vi "Priority Push.vi"(8 "error in (no error)":errorcluster, 10 "Action":T1, 11 "Subsystem in":refnum<queue>) -> (0 "error out":errorcluster, 3 "Subsystem out":refnum<queue>)   [LabVIEW 2014]
uses:
  Action/Action.ctl
  Action/Action Name.ctl
panel:
  out "Interrupted?":bool
  out "Ignored?":bool
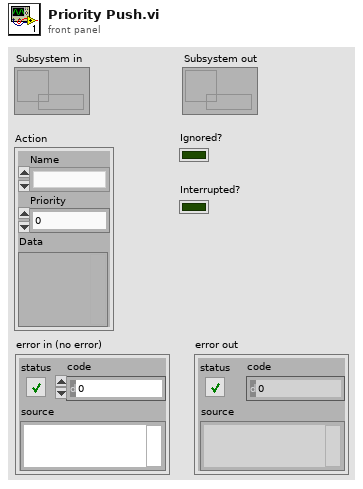
[diagram p1: front panel]
types:
  T1 = typedef "Action.ctl" = cluster{"Name":T2, "Priority":i32, "Data":variant}
  T2 = typedef "Action Name.ctl" = enum16{""}
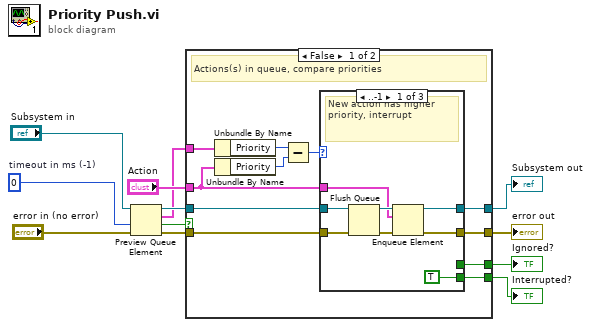
[diagram p0: block diagram]
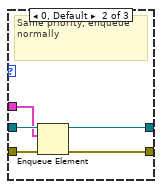
[diagram p2: hidden frame]
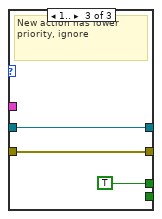
[diagram p3: hidden frame]
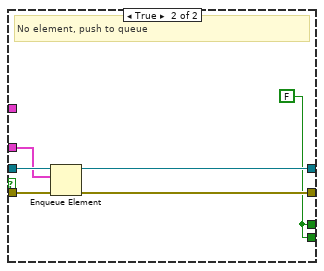
[diagram p4: hidden frame]
diagram:
  w11 = 0  # timeout in ms (-1)
  n1 = Preview Queue Element(queue="Subsystem in", timeout in ms (-1)=w11, error in (no error)="error in (no error)") -> (queue out=w9:refnum<queue>, element=w1:T1, timed out?=w10:bool, error out=w5:errorcluster)
  n2 = case shown="False" w10 {
    tunnel: w9 -> [w19 w45]
    tunnel: [w17 w44] -> w8
    tunnel: "Action" -> [w15 w43]
    tunnel: w5 -> [w18 w42]
    tunnel: [w16 w41] -> w4
    tunnel: [w14 w40] -> w3
    tunnel: [w13 w40] -> w2
    tunnel: w1 -> [w23 _]
    frame False {
      # "Actions(s) in queue, compare priorities"
      n3 = Unbundle By Name(w23) -> ("Priority"=w22:i32)
      n4 = Unbundle By Name(w15) -> ("Priority"=w21:i32)
      n5 = Subtract(x=w22, y=w21) -> (x-y=w20:i32)
      n6 = case shown="..-1" w20 {
        tunnel: w19 -> [w31 w36 w39]
        tunnel: w18 -> [w30 w34 w38]
        tunnel: [w29 w35 w39] -> w17
        tunnel: [w27 w33 w38] -> w16
        tunnel: w15 -> [w25 w32 _]
        tunnel: [_ _ TRUE] -> w14
        tunnel: [TRUE _ _] -> w13
        frame ..-1 {
          # "New action has higher priority, interrupt"
          n7 = Flush Queue(queue=w31, error in (no error)=w30) -> (queue out=w28:refnum<queue>, error out=w26:errorcluster)  [unwired: 1 out]
          n8 = Enqueue Element(queue=w28, element=w25, error in (no error)=w26) -> (queue out=w29:refnum<queue>, error out=w27:errorcluster)  [unwired: 1 in, 1 out]
        }
        frame 0, Default {
          # "Same priority, enqueue normally"
          n9 = Enqueue Element(queue=w36, element=w32, error in (no error)=w34) -> (queue out=w35:refnum<queue>, error out=w33:errorcluster)  [unwired: 1 in, 1 out]
        }
        frame 1.. {
          # "New action has lower priority, ignore"
        }
      }
    }
    frame True {
      w40 = FALSE
      # "No element, push to queue"
      n10 = Enqueue Element(queue=w45, element=w43, error in (no error)=w42) -> (queue out=w44:refnum<queue>, error out=w41:errorcluster)  [unwired: 1 in, 1 out]
    }
  }
  "error out" <- w4
  "Subsystem out" <- w8
  "Ignored?" <- w3
  "Interrupted?" <- w2
